vi "Tomography_v1.vi"() -> ()   [LabVIEW 2021]
uses:
  Ver_1/Config_File_Paths.ctl
  Ver_1/ZI_Data.ctl
  Ver_1/Cutted_Data.ctl
panel:
  in  "Save CYCLOPS data (?)":bool
  in  "Save raw data (?)":bool
  out "Measurement time [s]":dbl format="%.1f"
  out "single rot \nspectrum":waveform(dbl)[](graph)
  out "avg rot":cluster{"Time":dbl[], "X":dbl[]}[](graph)
  out "avg rot \nspectrum":waveform(dbl)[](graph)
  out "single rot":cluster{"Time":dbl[], "X":dbl[]}[](graph)
  out "single abs":cluster{"Time":dbl[], dbl[]}(graph)
  out "single differ":cluster{"Time":dbl[], "X":dbl[]}[](graph)
  out "Polarymeter":dbl(knob) scale=-15.0..15.0
  in  "Number of averages":u32=1 min=1 step=1
  out "loading":dbl(slide) scale=0.0..100.0
  in  "Resource Address":T1={"ZI Address"="DEV714", "VISA Keithley"="KEITHLEY", "VISA Arduino PG"="ARDUINO"}
  in  "Config files paths":T2={"ZI config file (.ini)"="Tomography_v1_config_dir\\Zurich_params.ini", "Keithley config file (.ini)"="Tomography_v1_config_dir\\Keithley_params.ini", "Arduino config file (.ini)"="Tomography_v1_config_dir\\pulse_sequence_dir\\"}
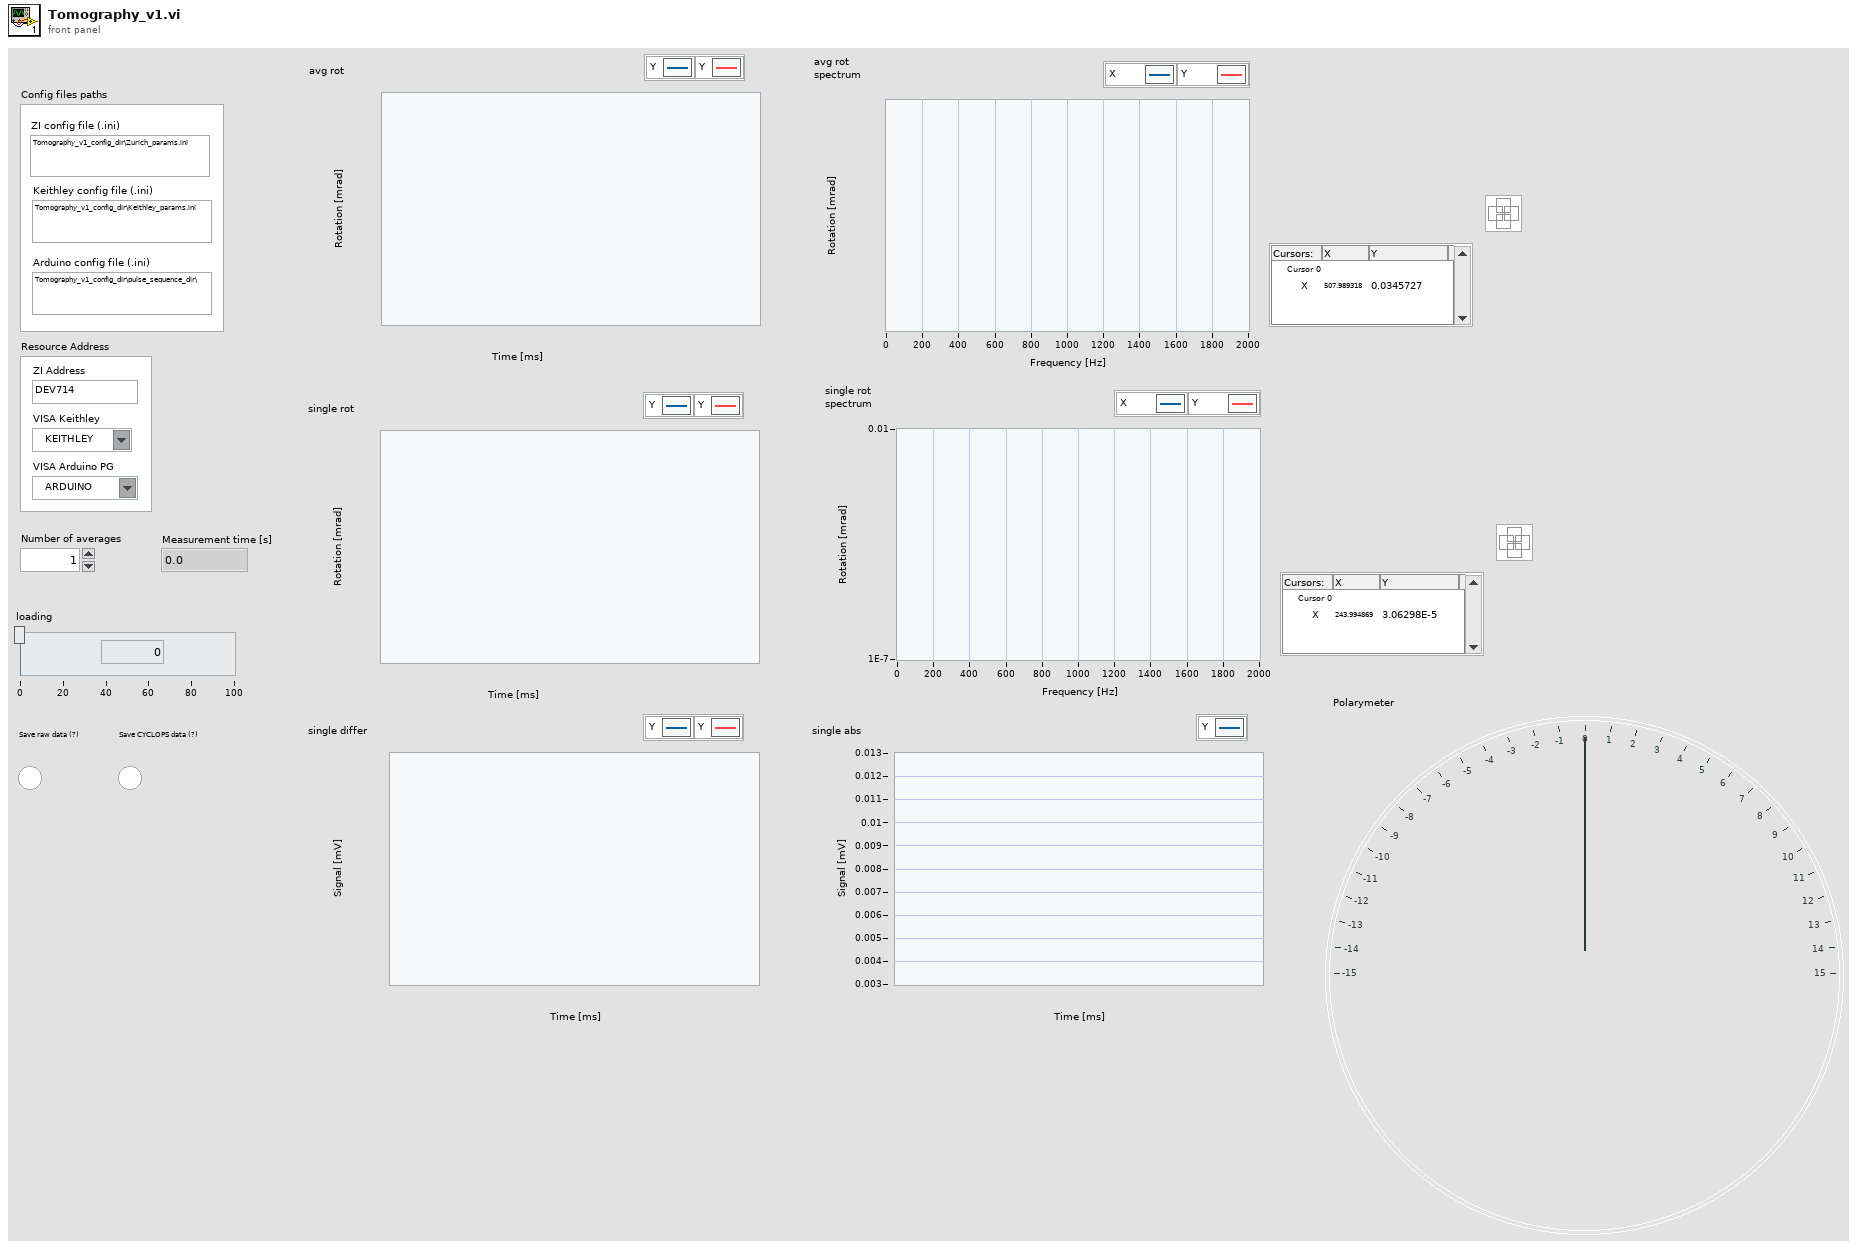
[diagram p1: front panel]
types:
  T1 = cluster{"ZI Address":string, "VISA Keithley":refnum<visa-resource-name>, "VISA Arduino PG":refnum<visa-resource-name>}
  T2 = typedef "Config_File_Paths.ctl" = cluster{"ZI config file (.ini)":string, "Keithley config file (.ini)":string, "Arduino config file (.ini)":string}
  T3 = typedef "ZI_Data.ctl" = cluster{"R":dbl[], "Theta":dbl[], "X":dbl[], "Y":dbl[], "AuxIn0":dbl[], "AuxIn1":dbl[], "Frequency":dbl[], "DIO":dbl[], "Time":dbl[]}
  T4 = typedef "Resources.ctl" = cluster{"ZI Handle":T5, "ZI ModHandle":T6, "VISA arduino":refnum<visa-resource-name>, "VISA Keithley":refnum<visa-resource-name>}
  T5 = typedef "Zurich Instruments LabOne.lvlib/ziTypeHandle.ctl" = cluster{"handleValid":bool, "Conn":u64, "Path Prefix":string, "Handle":u64, "Connected":bool, "Clockbase(s)":dbl}
  T6 = typedef "Zurich Instruments LabOne.lvlib/ziTypeModHandle.ctl" = cluster{"handleValid":bool, "Conn":u64, "ModHandle":u64, "moduleID":string, "Path Prefix":string}
  T7 = typedef "Cutted_Data.ctl" = cluster{"X":dbl[], "Y":dbl[], "Time":dbl[]}
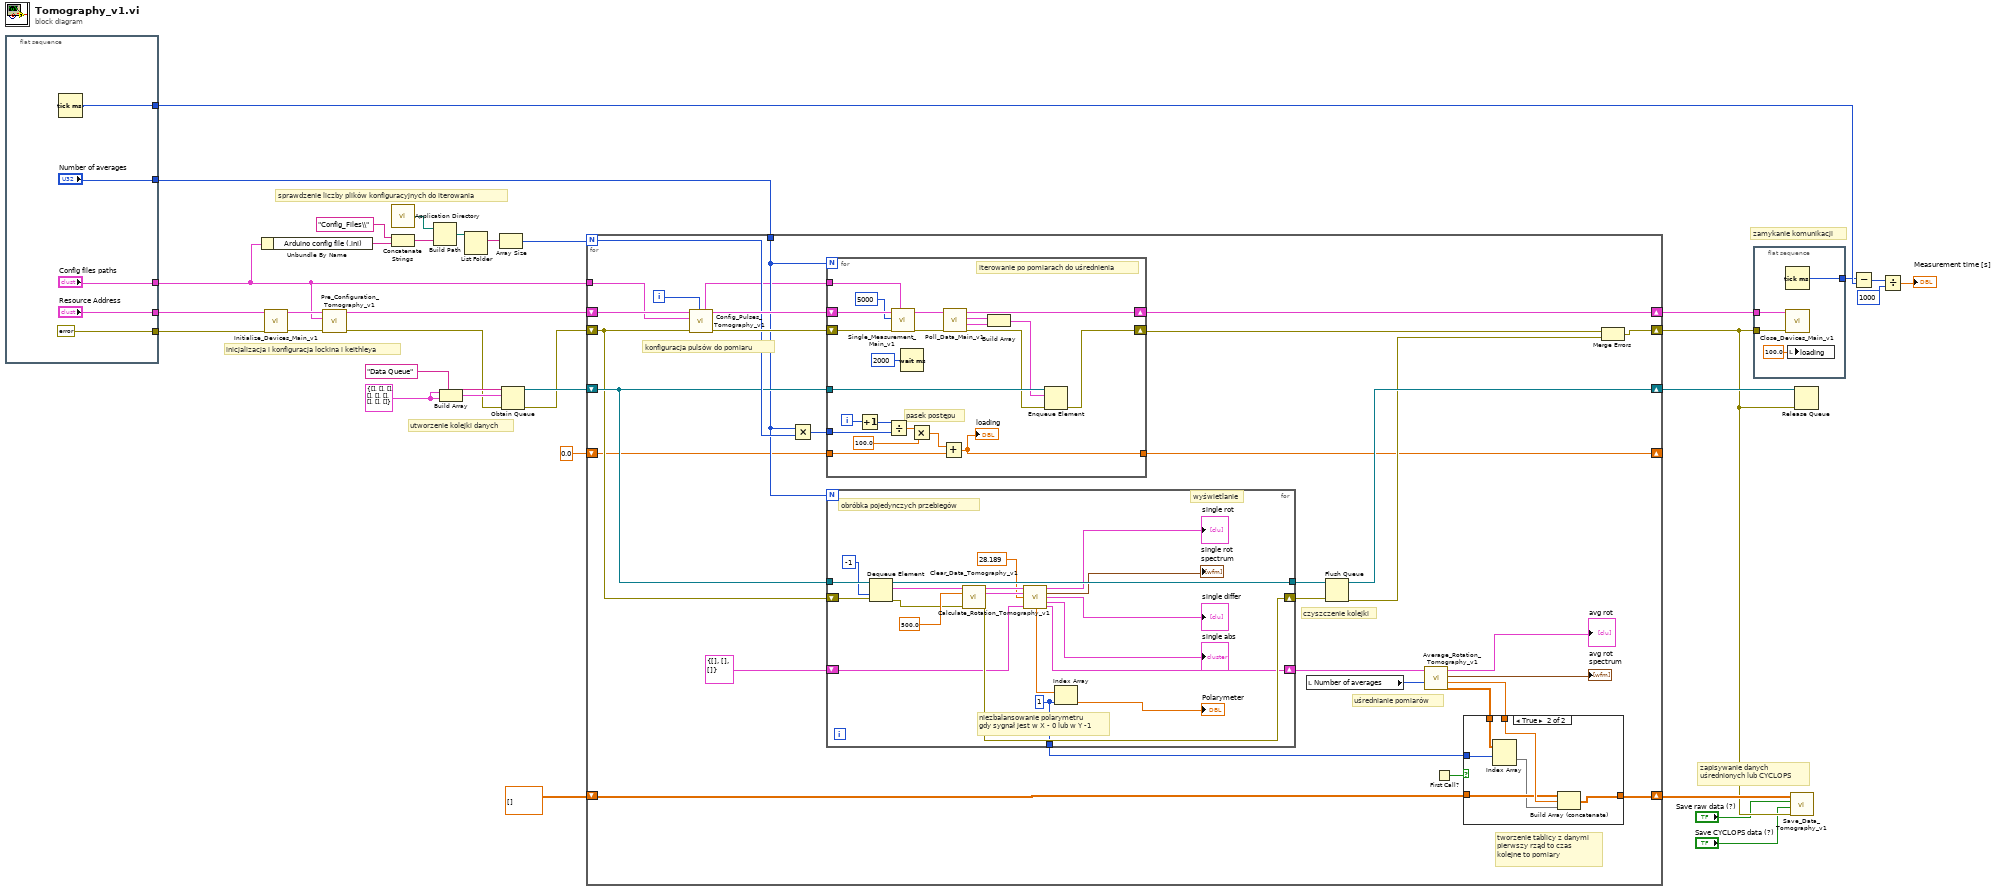
[diagram p0: block diagram]
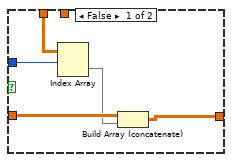
[diagram p2: hidden frame]
diagram:
  w18 = T3 {"R"=[], "Theta"=[], "X"=[], "Y"=[], "AuxIn0"=[], "AuxIn1"=[], "Frequency"=[], "DIO"=[], "Time"=[]} ("ZI Data")
  # "zapisywanie danych \nuśrednionych lub CYCLOPS"
  # "zamykanie komunikacji"
  # "utworzenie kolejki danych"
  # "sprawdzenie liczby plików konfiguracyjnych do iterowania"
  # "inicjalizacja i konfiguracja lockina i keithleya"
  n1 = flat-sequence {
    tunnel: ["Resource Address"] -> w31
    tunnel: [errorcluster {"status"=FALSE, "code"=0, "source"=""} ("error in")] -> w29
    tunnel: ["Config files paths"] -> w21
    tunnel: ["Number of averages"] -> w14
    tunnel: [w34] -> w10
    frame #0 {
      n2 = Tick Count (ms)() -> (millisecond timer value=w34:u32)
    }
  }
  n3 = Unbundle By Name(w21) -> ("Arduino config file (.ini)"=w27:string)
  n4 = call "Initialize_Devices_Main_v1.vi"("error in"=w29, "Resource Address"=w31) -> ("error out"=w32:errorcluster, "Resources"=w33:T4)  [unwired: 8 in]
  n5 = call "Pre_Configuration_Tomography_v1.vi"("error in"=w32, "Config files paths"=w21, "Resources in"=w33) -> ("error out"=w16:errorcluster, "Resources out"=w30:T4)  [unwired: 7 in]
  n6 = call <vilib>:"Application Directory.vi"() -> ("Application Directory"=w24:path)
  n7 = Concatenate Strings("Config_Files\\" ("string"), w27) -> (w28:string)
  n8 = Build Path(base path=w24, name or relative path=w28) -> (appended path=w25:path)
  n9 = Build Array(w18, w18) -> (w17:T3[])
  n10 = List Folder(path=w25) -> (filenames=w23:string[])  [unwired: 3 in, 3 out]
  n11 = Array Size(array=w23) -> (size(s)=w22:i32)
  n12 = Obtain Queue(name (unnamed)="Data Queue", element data type=w17, error in (no error)=w16) -> (queue out=w20:refnum<queue>, error out=w15:errorcluster)  [unwired: 2 in, 1 out]
  n13 = for {
    N: w22 -> [w63]
    shift-right: [w64] -> w12
    shift-left: w30 -> [w69]
    shift-right: [w44] -> w3
    shift-left: w15 -> [w60]
    tunnel: w21 -> [w65]
    shift-right: [w57] -> w13
    shift-left: w20 -> [w61]
    tunnel: w14 -> [w55]
    shift-right: [w45] -> w4
    shift-left: dbl[][] [] -> [w49]
    shift-right: [w39] -> _
    shift-left: 0.0 -> [w40]
    i -> [w68]
    # "czyszczenie kolejki"
    # "tworzenie tablicy z danymi\npierwszy rząd to czas\nkolejne to pomiary"
    # "uśrednianie pomiarów"
    # "konfiguracja pulsów do pomiaru"
    n14 = call "Config_Pulses_Tomography_v1.vi"("init file iterator"=w68, "error in"=w60, "Config files paths"=w65, "Resources in"=w69) -> ("error out"=w66:errorcluster, "Resources out"=w67:T4, "Config files paths (single)"=w41:T2)  [unwired: 3 in, 2 out]
    n15 = Multiply(x=w55, y=w63) -> (x*y=w62:u32)
    n16 = for {
      N: w55 -> [_]
      shift-right: [w112] -> w64
      shift-left: w67 -> [w120]
      shift-right: [w108] -> w43
      shift-left: w66 -> [w117]
      tunnel: w61 -> [w111]
      tunnel: w41 -> [w119]
      tunnel: w62 -> [w107]
      tunnel: w40 -> [w105]
      tunnel: [w104] -> w39
      i -> [w103]
      # "pasek postępu"
      # "iterowanie po pomiarach do uśrednienia"
      n17 = Increment(x=w103) -> (x+1=w102:i32)
      n18 = Divide(x=w102, y=w107) -> (x/y=w121:dbl)
      n19 = call "Single_Measurement_Main_v1.vi"("Config files paths"=w119, "error in"=w117, "Timeout [ms]"=u64 5000, "Resources In"=w120) -> ("error out"=w116:errorcluster, "Resources Out"=w118:T4)  [unwired: 6 in]
      n20 = Wait (ms)(milliseconds to wait=u32 2000) -> ()  [unwired: 1 out]
      n21 = Multiply(x=w121, y=100.0) -> (x*y=w106:dbl)
      n22 = Add(x=w106, y=w105) -> (x+y=w104:dbl)
      "loading" <- w104
      n23 = call "Poll_Data_Main_v1.vi"("error in"=w116, "Resources in"=w118) -> ("error out"=w109:errorcluster, "ZI Data 3"=w113:T3, "ZI Data 0"=w114:T3, "Resources out"=w112:T4)  [unwired: 6 in]
      n24 = Build Array(w114, w113) -> (w110:T3[])
      n25 = Enqueue Element(queue=w111, element=w110, error in (no error)=w109) -> (error out=w108:errorcluster)  [unwired: 1 in, 2 out]
    }
    n26 = for {
      N: w55 -> [_]
      tunnel: w61 -> [w100]
      shift-right: [w92] -> w58
      shift-left: w60 -> [w99]
      tunnel: [w97] -> w59
      shift-right: [w87] -> w54
      shift-left: T7 {"X"=[], "Y"=[], "Time"=[]} ("Cutted Data") -> [w89]
      tunnel: [w83] -> w46
      w83 = 1 ("index")
      # "wyświetlanie"
      # "obróbka pojedynczych przebiegów"
      # "niezbalansowanie polarymetru\ngdy sygnał jest w X - 0 lub w Y -1"
      n27 = Dequeue Element(queue=w100, timeout in ms (-1)=-1, error in (no error)=w99) -> (queue out=w97:refnum<queue>, element=w96:T3[], error out=w94:errorcluster)  [unwired: 1 out]
      n28 = call "Clear_Data_Tomography_v1.vi"("ZI Data 0/3"=w96, "Time Of Collected Data (ms)"=500.0, "error in"=w94) -> ("Cutted Data"=w91:T7, "Cutted Data 3"=w90:T7, "error out"=w92:errorcluster)  [unwired: 7 in, 3 out]
      n29 = call "Calculate_Rotation_Tomography_v1.vi"("Diff signal"=w91, "Sum signal"=w90, "Monitor to RF ratio"=28.189, "Summed data in"=w89) -> ("rotation signal"=→"single rot":cluster{"Time":dbl[], dbl[]}[], "rotation spectrum"=→"single rot \nspectrum":waveform(dbl)[], "differ signal"=→"single differ":cluster{"Time":dbl[], "Y":dbl[]}[], "absorption signal"=→"single abs":cluster{"Time":dbl[], dbl[]}, "Imbalance X/Y"=w88:dbl[], "Summed data out"=w87:T7)  [unwired: 6 in]
      n30 = Index Array(array=w88, index=w83) -> (element=→"Polarymeter":dbl)
    }
    n31 = local read "Number of averages"() -> (w53:u32)
    n32 = Flush Queue(queue=w59, error in (no error)=w58) -> (queue out=w57:refnum<queue>, error out=w42:errorcluster)  [unwired: 1 out]
    n33 = call "Average_Rotation_Tomography_v1.vi"("Number of averages"=w53, "Summed data"=w54) -> ("Data X/Y out"=w47:dbl[][], "Time"=w48:dbl[], "rotation spectrum"=→"avg rot \nspectrum":waveform(dbl)[], "rotation signal"=→"avg rot":cluster{"Time":dbl[], dbl[]}[])  [unwired: 6 in]
    n34 = First Call?() -> (First Call?: T/F=w50:bool)
    n35 = case shown="True" w50 {
      tunnel: w49 -> [w74 w77]
      tunnel: w48 -> [_ w78]
      tunnel: w47 -> [w72 w79]
      tunnel: w46 -> [w73 w80]
      tunnel: [w70 w75] -> w45
      frame False {
        n36 = Index Array(array=w72, index (row)=w73) -> (element=w71:dbl[])  [unwired: 1 in]
        n37 = Build Array (concatenate)(w74, w71) -> (w70:dbl[][])
      }
      frame True {
        n38 = Index Array(array=w79, index (row)=w80) -> (element=w76:dbl[])  [unwired: 1 in]
        n39 = Build Array (concatenate)(w77, w78, w76) -> (w75:dbl[][])
      }
    }
    n40 = Merge Errors(w43, w42) -> (w44:errorcluster)
  }
  n41 = flat-sequence {
    tunnel: w12 -> [w126]
    tunnel: w3 -> [w125]
    tunnel: [w124] -> w9
    frame #0 {
      n42 = Tick Count (ms)() -> (millisecond timer value=w124:u32)
      n43 = call "Close_Devices_Main_v1.vi"("error in"=w125, "Resources in"=w126) -> ()  [unwired: 9 in, 1 out]
      n44 = local write "loading"(100.0 ("loading")) -> ()
    }
  }
  n45 = call "Save_Data_Tomography_v1.vi"("error in"=w3, "Save CYCLOPS data (?)"="Save CYCLOPS data (?)", "Save raw data (?)"="Save raw data (?)", "Data Raw"=w4) -> ()  [unwired: 6 in, 2 out]
  n46 = Release Queue(queue=w13, error in (no error)=w3) -> ()  [unwired: 1 in, 3 out]
  n47 = Subtract(x=w9, y=w10) -> (x-y=w7:u32)
  n48 = Divide(x=w7, y=u32 1000) -> (x/y=→"Measurement time [s]":dbl)
